vi "存入mysql.vi"(7 "mysqldata簇":T1 {"JCSJ" format="%<%Y/%m/%d %H:%M:%S>T"}, 11 "table":string="t_sjzx_wryzxjc_fs_xssj") -> (3 "error out":errorcluster)   [LabVIEW 2016]
uses:
  <vilib>/addons/database/Connection.llb/DB Tools Open Connec (String).vi
  <vilib>/addons/database/NI_Database_API.lvlib
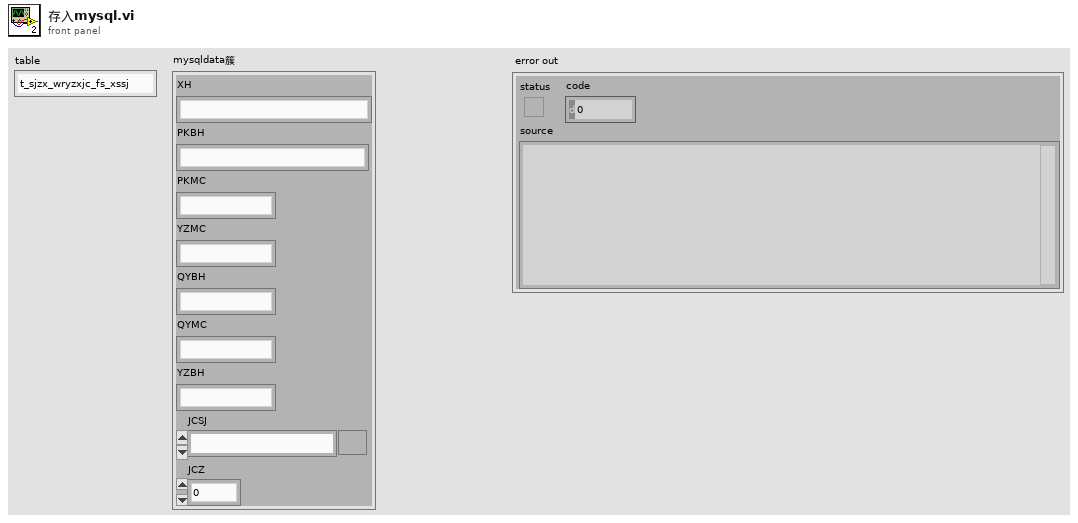
[diagram p1: front panel]
types:
  T1 = cluster{"XH":string, "PKBH":string, "PKMC":string, "YZMC":string, "QYBH":string, "QYMC":string, "YZBH":string, "JCSJ":timestamp, "JCZ":dbl}
  T2 = typedef "NI_Database_API.lvlib/Conn ObjectReference.ctl" = refnum<k1>
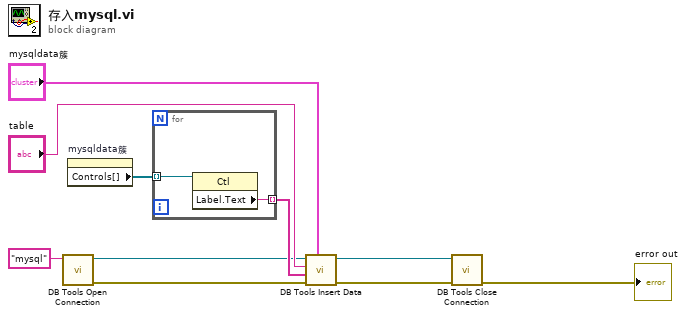
[diagram p0: block diagram]
diagram:
  n1 = call-poly <vilib>:"DB Tools Open Connection.vi"("connection information"="mysql") -> ("error out"=w1:errorcluster, "connection reference"=w2:T2)  [unwired: 7 in]
  n2 = property on="mysqldata簇" class="Clust (严格)"() -> ("Controls[]"=w5:refnum<vi>[])  [unwired: 2 in, 2 out]
  n3 = for {
    tunnel: w5 -> [w12] mode=indexing
    tunnel: [w11] -> w4 mode=indexing
    n4 = property class="Ctl"(reference=w12) -> ("Label.Text"=w11:string)  [unwired: 1 in, 2 out]
  }
  n5 = call <vilib>:"DB Tools Insert Data.vi"("data"="mysqldata簇", "error in (no error)"=w1, "columns"=w4, "table"="table", "connection reference"=w2) -> ("error out"=w8:errorcluster, "connection reference out"=w7:T2)  [unwired: 5 in]
  n6 = call <vilib>:"DB Tools Close Connection.vi"("error in (no error)"=w8, "connection reference"=w7) -> ("error out"=→"error out":errorcluster)  [unwired: 5 in]
